vi "Get Single Attribute.vi"(8 "error in (no error)":errorcluster, 9 "Data to get":refnum<class "Data.lvclass">, 10 "Name":string, 11 "Variant in":refnum<class "Variant.lvclass">) -> (0 "error out":errorcluster, 1 "Data out":refnum<class "Data.lvclass">, 2 "Found?":bool, 3 "Variant out":refnum<class "Variant.lvclass">)   [LabVIEW 2020, in "Data.lvlib" / "Variant.lvclass"]
doc: "Get a single attribute from the variant."
uses:
  Variant.lvclass
  Data.lvclass
  Variant.lvclass/Variant.ctl
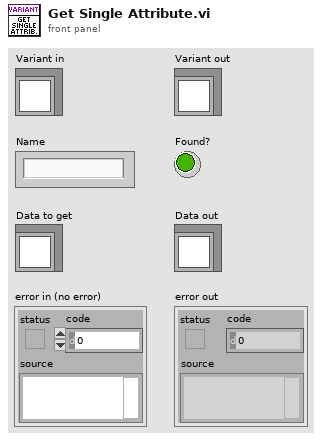
[diagram p1: front panel]
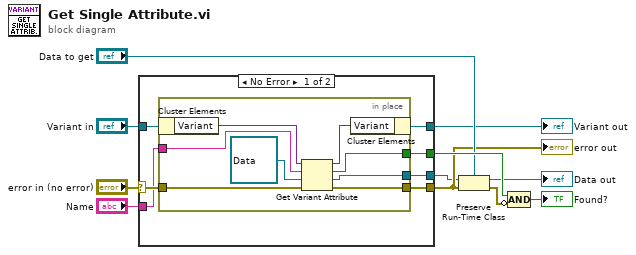
[diagram p0: block diagram]
diagram:
  n1 = case shown="No Error" "error in (no error)" {
    selector: "error in (no error)" -> [w16 w28]
    tunnel: [w15 w28] -> w4
    tunnel: [w17 w27] -> w3
    tunnel: "Variant in" -> [w18 w27]
    tunnel: "Name" -> [w14 _]
    tunnel: [w13 _] -> w8
    tunnel: [w12 _] -> w2
    frame No Error {
      n2 = in-place {
        in-place-border: w16 -> [w24]
        in-place-border: [w23] -> w15
        in-place-border: w14 -> [w22]
        in-place-border: [w21] -> w13
        in-place-border: [w19] -> w12
        n3 = in-place-cluster #1(w18) -> ("Variant"=w26:variant)
        n4 = Get Variant Attribute(Variant=w26, name=w22, default value (empty Variant)=refnum<class "Data.lvclass"> refnum ("Data.lvlib:Data.lvclass"), error in=w24) -> (duplicate Variant=w25:variant, found=w21:bool, value=w19:refnum<class "Data.lvclass">, error out=w23:errorcluster)
        n5 = in-place-cluster #1("Variant"=w25) -> (w17:refnum<class "Variant.lvclass">)
      }
    }
    frame Error {
    }
  }
  "error out" <- w4
  "Variant out" <- w3
  n6 = Preserve Run-Time Class(object in=w2, error in=w4, 2:"Data to get") -> (object out=→"Data out":refnum<class "Data.lvclass">, error out=w5:errorcluster)
  n7 = Compound Arithmetic op=AND(w8, invert w5) -> (→"Found?":bool)
